vi "PI Goto GPIB.vi"(0 "System no.":i32=1 min=1 max=4 step=1, 1 "x-position":dbl format="%.2f", 2 "y-position":dbl format="%.2f", 3 "z-position":dbl, 5 "error in":errorcluster) -> (19 "error out":errorcluster)   [LabVIEW 2013]
doc: "This VI checks if the connection to the selected system is already open and, if it is, it closes this connection. \n\nValid for C-843, C-843.PM, C-844, C-865, E-710 (but must be present in Communication.llb for all other systems, too)"
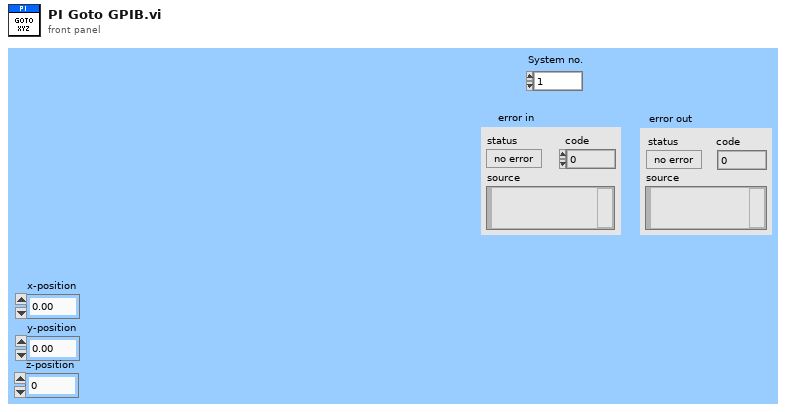
[diagram p1: front panel]
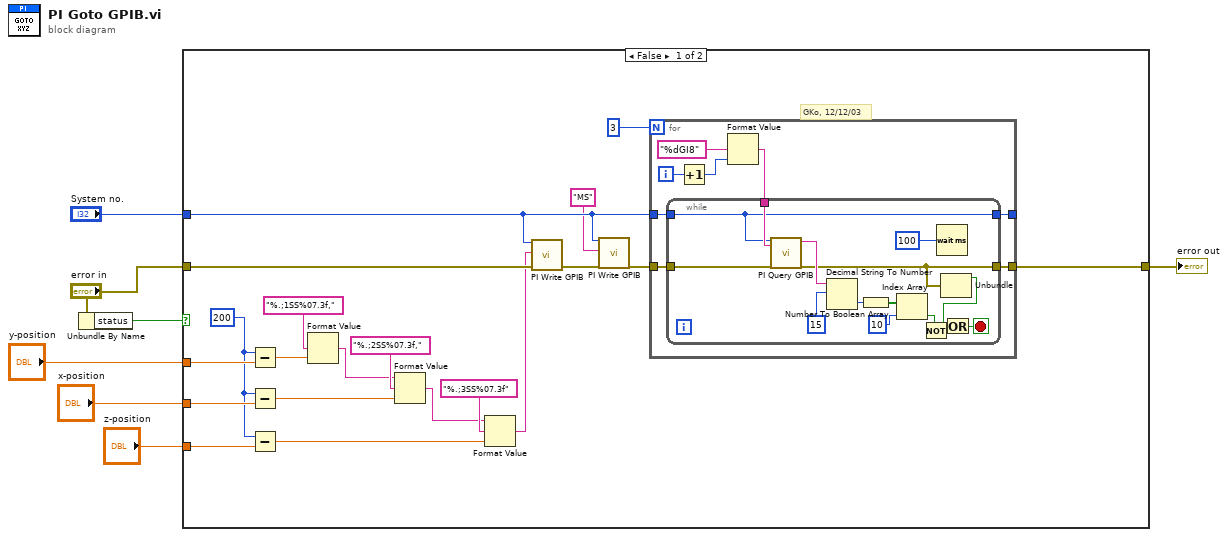
[diagram p0: block diagram]
diagram:
  # "GKo, 12/12/03"
  n1 = Unbundle By Name("error in") -> ("status"=w4:bool)
  n2 = case shown="False" w4 {
    tunnel: "System no." -> [w13 _]
    tunnel: "error in" -> [w15 w50]
    tunnel: [w11 w50] -> w6
    tunnel: "z-position" -> [w27 _]
    tunnel: "x-position" -> [w26 _]
    tunnel: "y-position" -> [w25 _]
    frame False {
      w24 = 200
      n3 = Subtract(x=w24, y=w25) -> (x-y=w23:dbl)
      n4 = Subtract(x=w24, y=w26) -> (x-y=w19:dbl)
      n5 = Subtract(x=w24, y=w27) -> (x-y=w17:dbl)
      n6 = Format Value(format string="%.;1SS%07.3f,", value (0)=w23) -> (output string=w18:string)  [unwired: 1 in]
      n7 = Format Value(string ("")=w18, format string="%.;2SS%07.3f,", value (0)=w19) -> (output string=w16:string)
      n8 = Format Value(string ("")=w16, format string="%.;3SS%07.3f", value (0)=w17) -> (output string=w9:string)
      n9 = call "PI Write GPIB.vi"("System no."=w13, "String to send"=w9, "error in"=w15) -> ("error out"=w14:errorcluster)  [unwired: 16 in]
      n10 = call "PI Write GPIB.vi"("System no."=w13, "String to send"="MS", "error in"=w14) -> ("error out"=w12:errorcluster)  [unwired: 16 in]
      n11 = for {
        N: 3 -> [_]
        tunnel: w12 -> [w31]
        tunnel: w13 -> [w30]
        tunnel: [w29] -> w11
        tunnel: [w28] -> _
        i -> [w35]
        n12 = Increment(x=w35) -> (x+1=w34:i32)
        n13 = Format Value(format string="%dGI8", value (0)=w34) -> (output string=w32:string)  [unwired: 1 in]
        n14 = while {
          tunnel: w32 -> [w49]
          tunnel: w31 -> [w48]
          tunnel: w30 -> [w44]
          tunnel: [w43] -> w29
          tunnel: [w44] -> w28
          stop <- w38 stop-if-true
          n15 = call "PI Query GPIB.vi"("System no."=w44, "String to send"=w49, "error in"=w48) -> ("String read"=w46:string, "error out"=w43:errorcluster)  [unwired: 14 in, 1 out]
          n16 = Decimal String To Number(string=w46, offset=15) -> (number=w45:i32)  [unwired: 1 in, 1 out]
          n17 = Number To Boolean Array(number=w45) -> (Boolean array=w40:bool[])
          n18 = Index Array(array=w40, index=10) -> (element=w39:bool)
          n19 = Not(x=w39) -> (.not. x?=w36:bool)
          n20 = Wait (ms)(milliseconds to wait=100) -> ()  [unwired: 1 out]
          n21 = Unbundle(w43) -> ("status"=w42:bool)  [unwired: 2 out]
          n22 = Or(x=w42, y=w36) -> (x .or. y?=w38:bool)
        }
      }
    }
    frame True {
    }
  }
  "error out" <- w6
